vi "Create.vi"(5 "Default Control Behavior":T1, 7 "VI Reference":refnum<vi>, 8 "error in (no error)":errorcluster, 9 "VI Name":string, 10 "Show Config Dialog":bool=TRUE, 11 "Web FP In":refnum<class "Web Front Panel.lvclass">) -> (0 "error out":errorcluster, 3 "Web FP Out":refnum<class "Web Front Panel.lvclass">)   [LabVIEW 2015, in "Front Panel Publisher.lvlib" / "Web Front Panel.lvclass"]
uses:
  Web Front Panel.lvclass
  Controls/Cluster - Default Control Behavior.ctl
  Front Panel Objects/Object_class/Object.lvclass
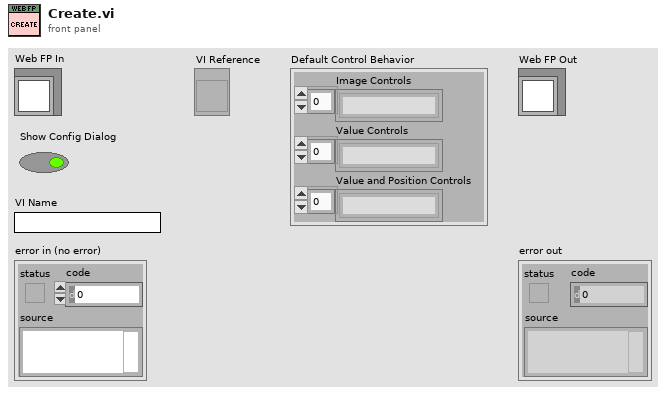
[diagram p1: front panel]
types:
  T1 = typedef "Front Panel Publisher.lvlib/Web Front Panel.lvclass/Cluster - Default Control Behavior.ctl" = cluster{"Image Controls":string[], "Value Controls":string[], "Value and Position Controls":string[]}
  T2 = typedef "LVPointTypeDef.ctl" = cluster{"Horizontal":i16, "Vertical":i16}
  T3 = typedef "Front Panel Publisher.lvlib/Web Front Panel.lvclass/Object Attributes.ctl" = cluster{"VI Name":string, "VI Reference":refnum<vi>, "Controls":refnum<class "Object.lvclass">[], "Indicators":refnum<class "Object.lvclass">[], "Decorations":refnum<class "Object.lvclass">[], "VR With Previous Get":refnum<data-value>, "VR With Ring Images":refnum<data-value>, "Panel Origin":T2}
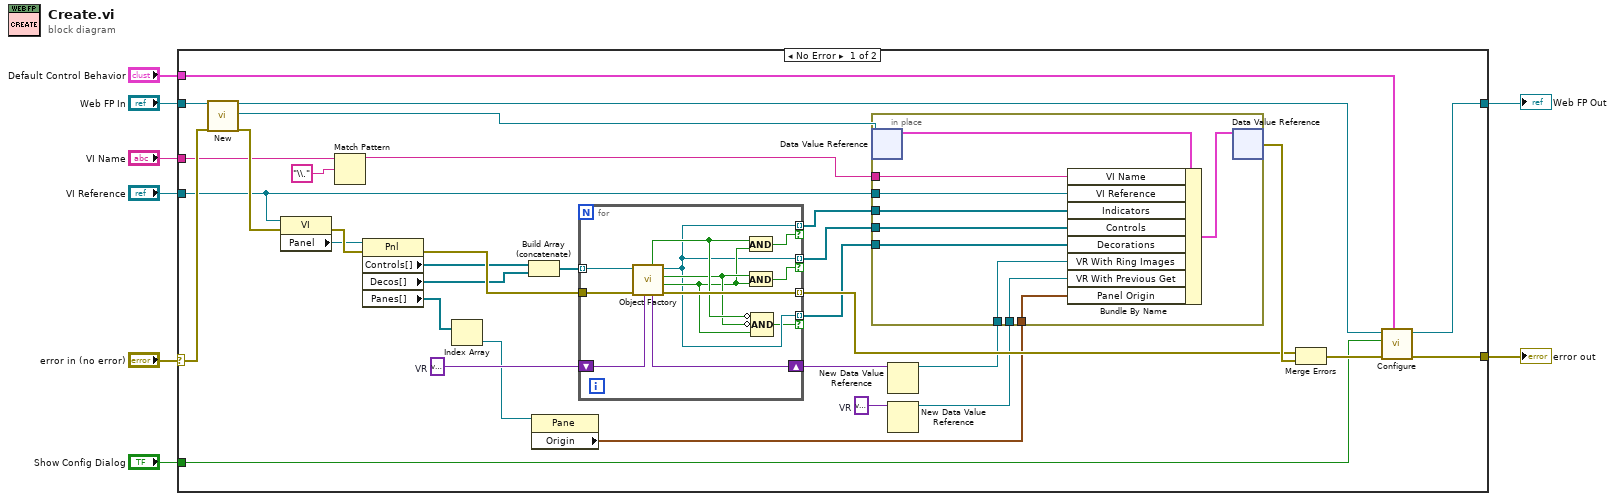
[diagram p0: block diagram]
diagram:
  n1 = case shown="No Error" "error in (no error)" {
    selector: "error in (no error)" -> [w41 w65]
    tunnel: [w27 w65] -> w7
    tunnel: "Web FP In" -> [w36 w64]
    tunnel: [w14 w64] -> w5
    tunnel: "VI Name" -> [w30 _]
    tunnel: "VI Reference" -> [w34 _]
    tunnel: "Show Config Dialog" -> [w24 _]
    tunnel: "Default Control Behavior" -> [w16 _]
    frame No Error {
      w23 = variant  # VR
      w26 = variant  # VR
      n2 = call "New.vi"("Web FP In"=w36, "error in (no error)"=w41) -> ("Web FP Out"=w15:refnum<class "Web Front Panel.lvclass">, "DVRRefOut"=w35:refnum<data-value>, "error out"=w39:errorcluster)  [unwired: 14 in, 1 out]
      n3 = property class="VI"(reference=w34, error in=w39) -> (error out=w37:errorcluster, "Panel"=w13:refnum<vi>)  [unwired: 1 out]
      n4 = Match Pattern(string=w30, regular expression="\\.") -> (before substring=w29:string)  [unwired: 1 in, 3 out]
      n5 = property class="Pnl"(reference=w13, error in=w37) -> (error out=w38:errorcluster, "Controls[]"=w33:refnum<vi>[], "Decos[]"=w12:refnum<vi>[], "Panes[]"=w11:refnum<vi>[])  [unwired: 1 out]
      n6 = Index Array(array=w11) -> (element=w10:refnum<vi>)  [unwired: 1 in]
      n7 = Build Array (concatenate)(w33, w12) -> (w20:refnum<vi>[])
      n8 = property class="Pane"(reference=w10) -> ("Origin"=w9:T2)  [unwired: 1 in, 2 out]
      n9 = for {
        tunnel: w20 -> [w51] mode=indexing
        tunnel: [w44] -> w17 mode=indexing if=w50
        tunnel: [w44] -> w18 mode=indexing if=w49
        tunnel: w38 -> [w53]
        tunnel: [w52] -> w32 mode=indexing
        shift-right: [w48] -> w22
        shift-left: w23 -> [w42]
        tunnel: [w44] -> w19 mode=indexing if=w43
        n10 = call "Object Factory.vi"("Ring Images In"=w42, "error in (no error)"=w53, "GOject In"=w51) -> ("error out"=w52:errorcluster, "Is Visible"=w45:bool, "Is Control"=w46:bool, "Object Out"=w44:refnum<class "Object.lvclass">, "Ring Images Out"=w48:variant, "Is Indicator"=w47:bool)  [unwired: 3 in]
        n11 = And(x=w47, y=w45) -> (x .and. y?=w50:bool)
        n12 = And(x=w46, y=w45) -> (x .and. y?=w49:bool)
        n13 = Compound Arithmetic op=AND(invert w47, invert w46, w45) -> (w43:bool)
      }
      n14 = New Data Value Reference(data value=w22) -> (data value reference=w21:refnum<data-value>)  [unwired: 1 in, 1 out]
      n15 = New Data Value Reference(data value=w26) -> (data value reference=w25:refnum<data-value>)  [unwired: 1 in, 1 out]
      n16 = in-place {
        in-place-border: w29 -> [w61]
        in-place-border: w34 -> [w60]
        in-place-border: w17 -> [w59]
        in-place-border: w18 -> [w58]
        in-place-border: w19 -> [w57]
        in-place-border: w25 -> [w56]
        in-place-border: w21 -> [w55]
        in-place-border: w9 -> [w54]
        n17 = in-place-dvr #1(w35) -> (w62:T3)  [unwired: 1 out]
        n18 = Bundle By Name(cluster=w62, "VI Name"=w61, "VI Reference"=w60, "Indicators"=w59, "Controls"=w58, "Decorations"=w57, "VR With Ring Images"=w55, "VR With Previous Get"=w56, "Panel Origin"=w54) -> (w63:T3)
        n19 = in-place-dvr #1(w63) -> (w40:errorcluster)  [unwired: 1 out]
      }
      n20 = Merge Errors(w32, w40) -> (w28:errorcluster)
      n21 = call "Configure.vi"("Default Control Behavior"=w16, "error in (no error)"=w28, "Show Config"=w24, "reference in"=w15) -> ("error out"=w27:errorcluster, "reference out"=w14:refnum<class "Web Front Panel.lvclass">)  [unwired: 6 in]
    }
    frame Error {
    }
  }
  "error out" <- w7
  "Web FP Out" <- w5
